vi "计算结果-步响应-伸出实测.vi"(3 "步响应计算参数 in":T2, 4 "步响应控制参数 in":T1={"rise_step"=1.0, "rise_criterion"=600.0, "peak_step"=1.0, "peak_criterion"=50.0, "nb_of_peaks"=200.0}, 5 "行程 in":dbl[](array[numeric])) -> (0 "步响应计算参数 out":T2, 1 "步响应控制参数 out":T1={"rise_step"=1.0, "rise_criterion"=600.0, "peak_step"=1.0, "peak_criterion"=50.0, "nb_of_peaks"=200.0}, 2 "行程 out":dbl[](array[numeric]))   [LabVIEW 2013]
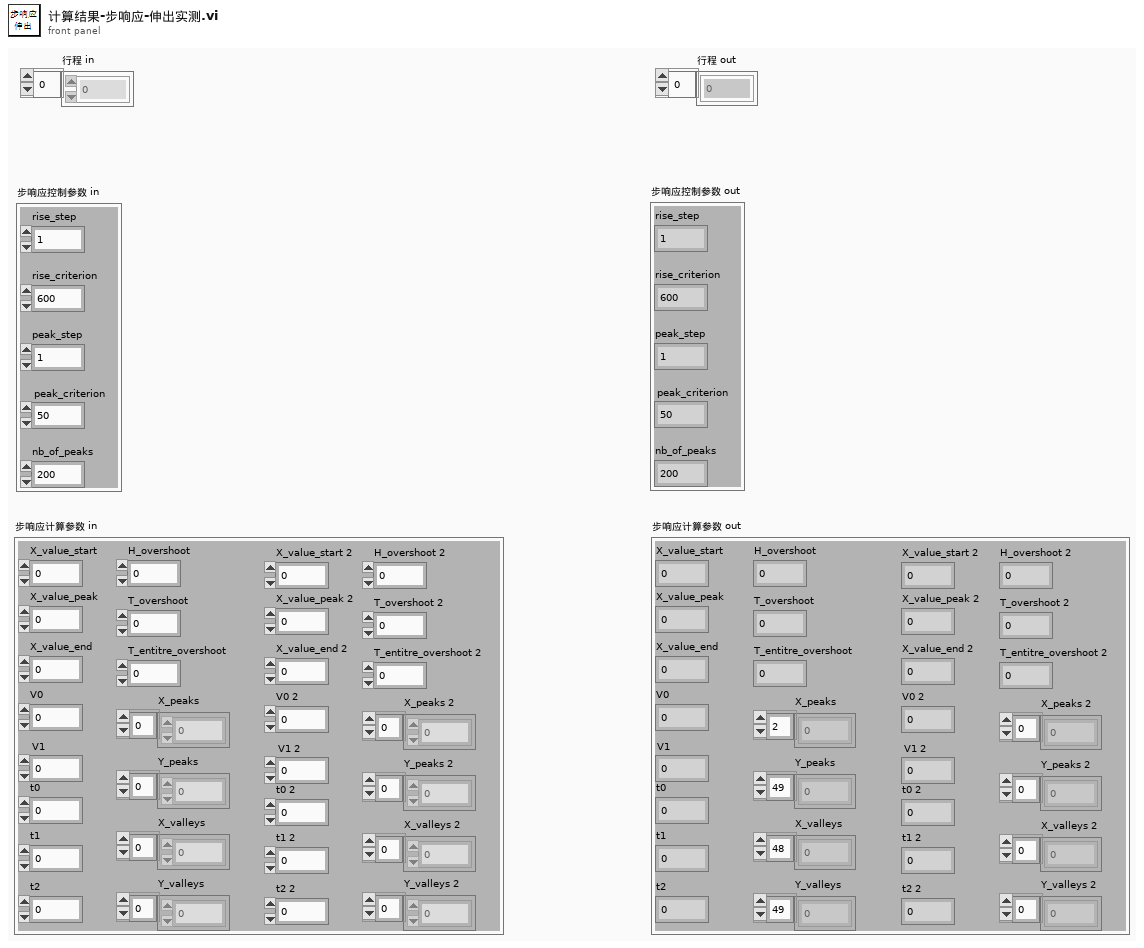
[diagram p1: front panel]
types:
  T1 = cluster{"rise_step":dbl, "rise_criterion":dbl, "peak_step":dbl, "peak_criterion":dbl, "nb_of_peaks":dbl}
  T2 = cluster{"X_value_start":dbl, "X_value_peak":dbl, "t1":dbl, "X_value_end":dbl, "V0":dbl, "V1":dbl, "t0":dbl, "X_peaks":dbl[], "X_valleys":dbl[], "Y_peaks":dbl[], "Y_valleys":dbl[], "t2":dbl, "H_overshoot":dbl, "T_overshoot":dbl, "T_entitre_overshoot":dbl, "X_value_start 2":dbl, "X_value_peak 2":dbl, "t1 2":dbl, "X_value_end 2":dbl, "V0 2":dbl, "V1 2":dbl, "t0 2":dbl, "X_peaks 2":dbl[], "X_valleys 2":dbl[], "Y_peaks 2":dbl[], "t2 2":dbl, "H_overshoot 2":dbl, "T_overshoot 2":dbl, "T_entitre_overshoot 2":dbl, "Y_valleys 2":dbl[]}
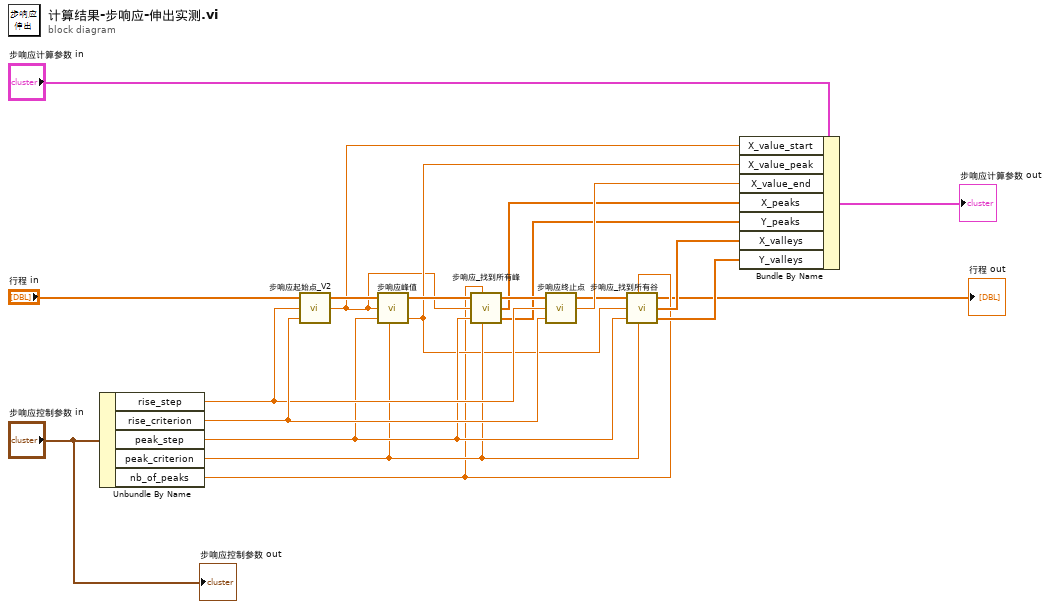
[diagram p0: block diagram]
diagram:
  n1 = Unbundle By Name("步响应控制参数 in") -> ("rise_step"=w16:dbl, "rise_criterion"=w17:dbl, "peak_step"=w15:dbl, "peak_criterion"=w14:dbl, "nb_of_peaks"=w4:dbl)
  n2 = call "步响应起始点_V2.vi"("（要求）连续大于0的次数"=w17, "rise_step"=w16, "行程 in"="行程 in") -> ("X_value"=w5:dbl, "行程 out"=w21:dbl[])  [unwired: 1 in]
  n3 = call "步响应峰值.vi"("行程 in"=w21, "X_start"=w5, "peak_step"=w15, "（要求）连续大于0的次数"=w14) -> ("行程 out"=w20:dbl[], "X_value_next"=w6:dbl)  [unwired: 1 in, 1 out]
  n4 = call "步响应_找到所有峰.vi"("行程 in"=w20, "nb_of_peaks"=w4, "X_peak_start"=w5, "step_peak"=w15, "（要求）连续大于0的次数"=w14) -> ("行程 out"=w19:dbl[], "X_Peaks"=w9:dbl[], "Y_Peaks"=w8:dbl[])
  n5 = call "步响应终止点.vi"("（要求）连续大于0的次数"=w17, "step"=w16, "行程 in"=w19) -> ("X_value"=w10:dbl, "行程 out"=w7:dbl[])  [unwired: 1 in]
  n6 = call "步响应_找到所有谷.vi"("行程 in"=w7, "nb_of_peaks"=w4, "X_valley_start"=w6, "step_valley"=w15, "（要求）连续大于0的次数"=w14) -> ("行程 out"=→"行程 out":dbl[], "X_valley"=w12:dbl[], "Y_valley"=w11:dbl[])
  n7 = Bundle By Name(cluster="步响应计算参数 in", "X_value_start"=w5, "X_value_peak"=w6, "X_value_end"=w10, "X_peaks"=w9, "Y_peaks"=w8, "X_valleys"=w12, "Y_valleys"=w11) -> (→"步响应计算参数 out":T2)
  "步响应控制参数 out" <- "步响应控制参数 in"
